vi "HardSafety.vi"(0 "Safety Been Triggered":bool, 3 "Potentiometers":dbl[](array[numeric]), 4 "Position From Rot Encoder":dbl, 6 "Force Sensor Faulty":bool, 7 "Pots Diff Too Much At Init":bool, 8 "LY":dbl, 9 "LX":dbl, 10 "RY":dbl, 11 "RX":dbl) -> (2 "HARD SAFETY":bool)   [LabVIEW 2019]
panel:
  out "Rot Pot":bool
  out "Rot Potentiometers and Rot encoder too different":bool
  out "LY @ Trig":dbl
  out "RY @ Trig":dbl
  out "LX @ Trig":dbl
  out "RX @ Trig":dbl
  out "Y force":bool
  out "X force":bool
  out "Lin Potentiometers and Lin encoder too different":bool
  out "Y Force Diff Too Much":bool
  out "X Force Diff Too Much":bool
  # "At trigger"
  # "Forces"
  # "Potentiometers"
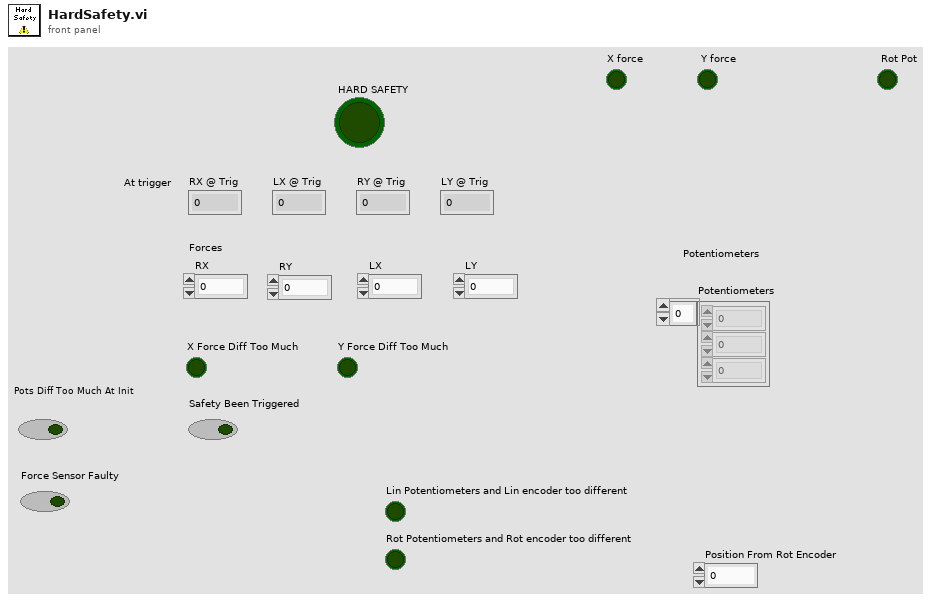
[diagram p1: front panel]
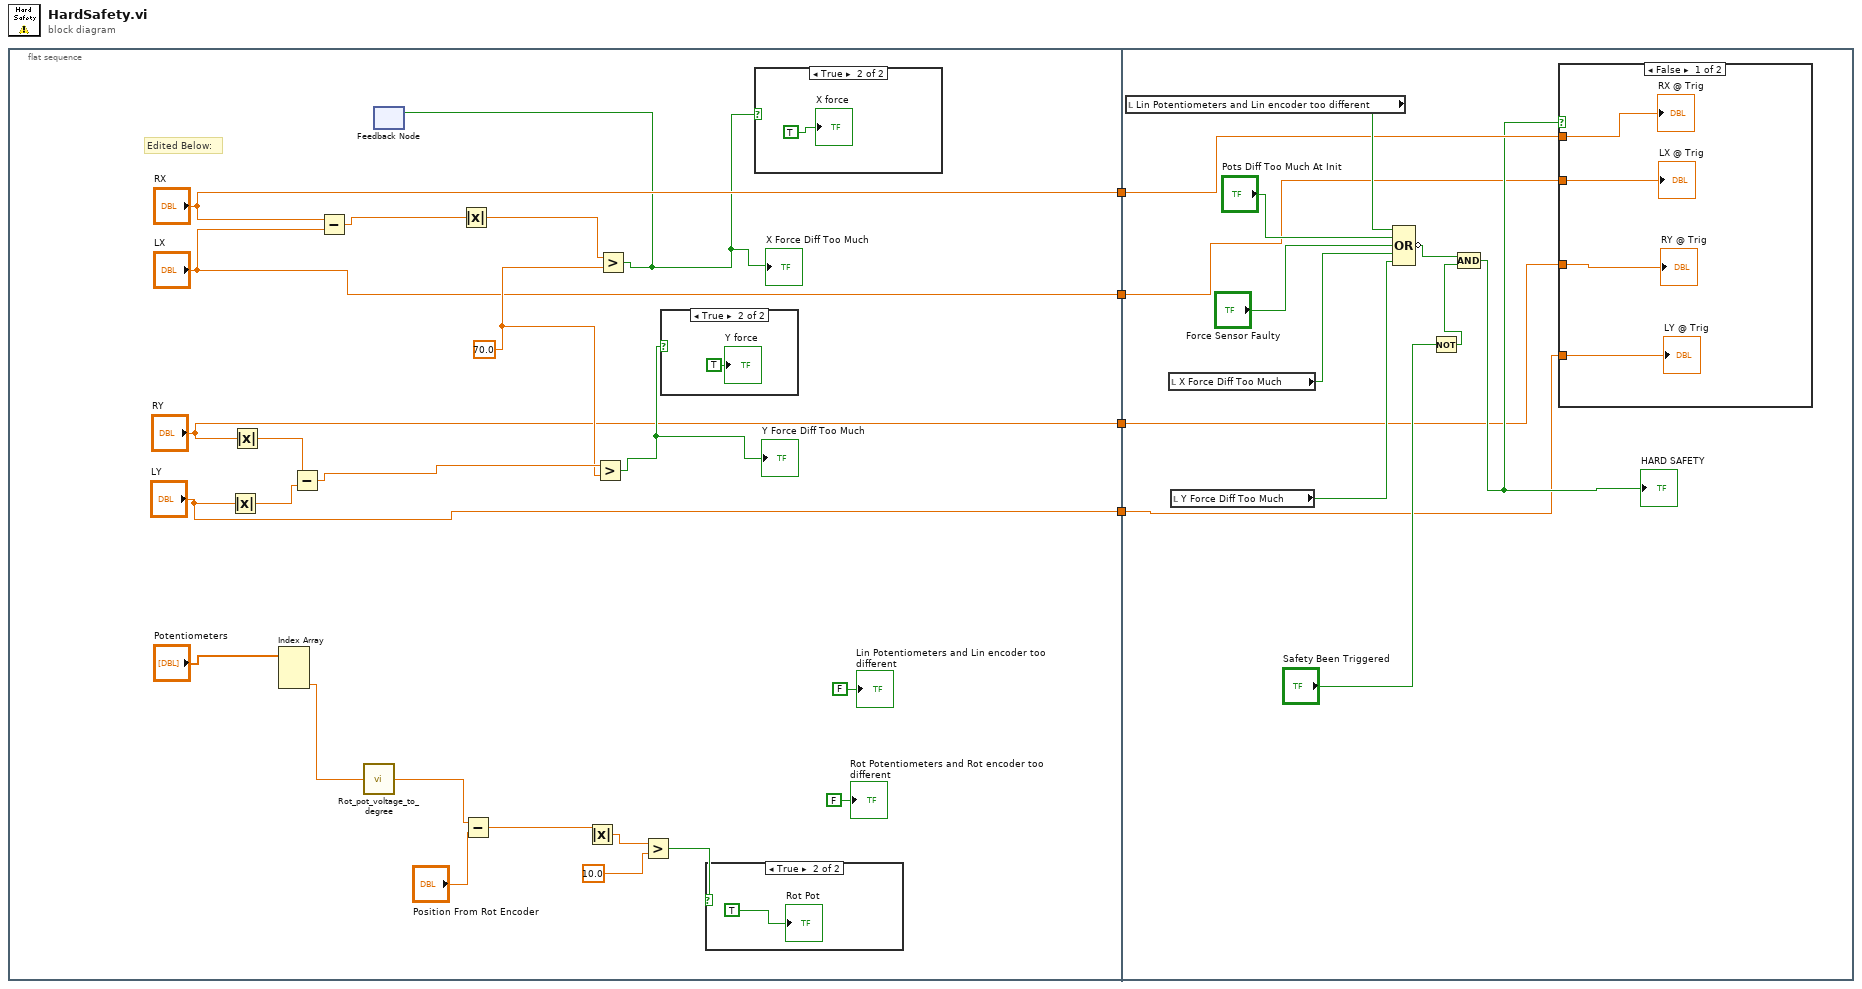
[diagram p0: block diagram]
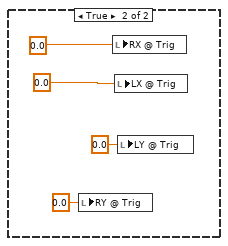
[diagram p5: hidden frame]
diagram:
  n1 = flat-sequence {
    tunnel: ["RX"] -> w4
    tunnel: ["LX"] -> w3
    tunnel: ["RY"] -> w2
    tunnel: ["LY"] -> w1
    tunnel: w4 -> [w34]
    tunnel: w3 -> [w32]
    tunnel: w2 -> [w31]
    tunnel: w1 -> [w30]
    frame #0 {
      w21 = 70.0
      # "Edited Below:"
      n2 = Absolute Value(x="LY") -> (abs(x)=w23:dbl)
      n3 = Absolute Value(x="RY") -> (abs(x)=w24:dbl)
      n4 = Index Array(array="Potentiometers") -> (element #3=w13:dbl)  [unwired: 3 in, 2 out]
      n5 = Subtract(x=w24, y=w23) -> (x-y=w22:dbl)
      n6 = Subtract(x="RX", y="LX") -> (x-y=w26:dbl)
      n7 = call "Rot_pot_voltage_to_degree.vi"("RotaryPot (Voltage)"=w13) -> ("RotaryPot (degree)"=w12:dbl)
      n8 = feedback #1() -> ()  [unwired: 2 in]
      n9 = Absolute Value(x=w26) -> (abs(x)=w25:dbl)
      n10 = Subtract(x=w12, y="Position From Rot Encoder") -> (x-y=w8:dbl)
      n11 = Absolute Value(x=w8) -> (abs(x)=w10:dbl)
      n12 = Greater?(x=w22, y=w21) -> (0:w19:bool)
      "Y Force Diff Too Much" <- w19
      n13 = Greater?(x=w25, y=w21) -> (0:w14:bool)
      "X Force Diff Too Much" <- w14
      n14 = feedback-in #1(w14) -> ()
      n15 = Greater?(x=w10, y=10.0) -> (0:w7:bool)
      n16 = case shown="True" w19 {
        frame False {
        }
        frame True {
          "Y force" <- TRUE ("Boolean 2")
        }
      }
      n17 = case shown="True" w7 {
        frame False {
        }
        frame True {
          "Rot Pot" <- TRUE ("Boolean 3")
        }
      }
      n18 = case shown="True" w14 {
        frame False {
        }
        frame True {
          "X force" <- TRUE
        }
      }
      "Lin Potentiometers and Lin encoder too different" <- FALSE ("Lin Potentiometers and Lin encoder too different")
      "Rot Potentiometers and Rot encoder too different" <- FALSE ("Rot Potentiometers and Rot encoder too different")
    }
    frame #1 {
      n19 = local read "Lin Potentiometers and Lin encoder too different"() -> (w36:bool)
      n20 = local read "X Force Diff Too Much"() -> (w38:bool)
      n21 = local read "Y Force Diff Too Much"() -> (w37:bool)
      n22 = Compound Arithmetic op=OR(w36, "Pots Diff Too Much At Init", "Force Sensor Faulty", w38, w37) -> (invert w35:bool)
      n23 = Not(x="Safety Been Triggered") -> (.not. x?=w39:bool)
      n24 = Compound Arithmetic op=AND(w35, w39) -> (w33:bool)
      "HARD SAFETY" <- w33
      n25 = case shown="False" w33 {
        tunnel: w34 -> [w46 _]
        tunnel: w32 -> [w45 _]
        tunnel: w31 -> [w44 _]
        tunnel: w30 -> [w43 _]
        frame False {
          "RX @ Trig" <- w46
          "LX @ Trig" <- w45
          "RY @ Trig" <- w44
          "LY @ Trig" <- w43
        }
        frame True {
          n26 = local write "RY @ Trig"(0.0 ("RY @ Trig")) -> ()
          n27 = local write "RX @ Trig"(0.0 ("RX")) -> ()
          n28 = local write "LX @ Trig"(0.0 ("LX @ Trig")) -> ()
          n29 = local write "LY @ Trig"(0.0 ("LY @ Trig")) -> ()
        }
      }
    }
  }
